vi "Mappatura registri.vi"() -> (3 "Mappa registri":string[][](array[string]))   [LabVIEW 2019]
uses:
  <vilib>/Utility/file.llb/Read From Spreadsheet File (string).vi
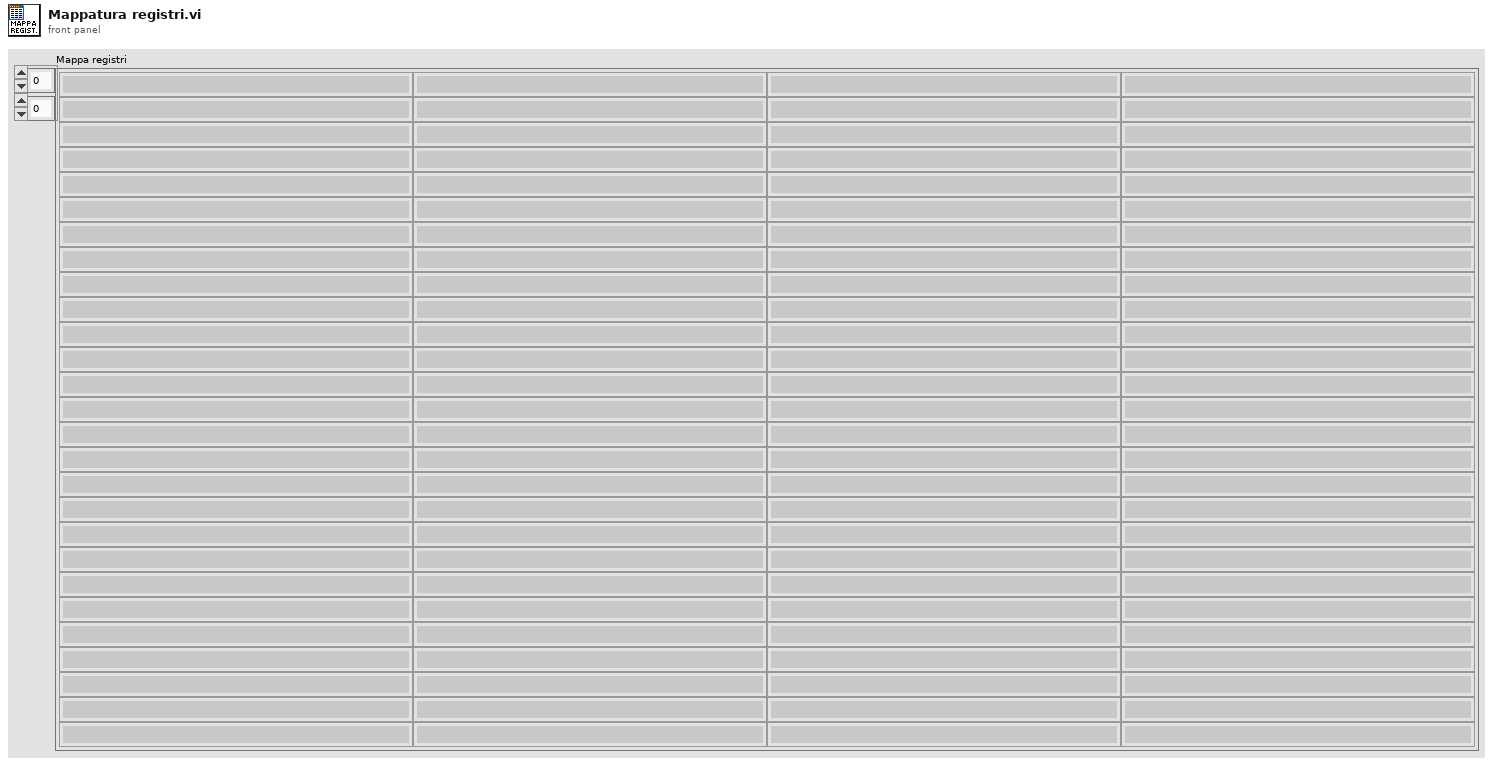
[diagram p1: front panel]
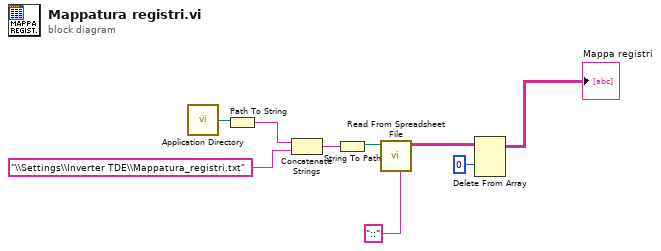
[diagram p0: block diagram]
diagram:
  n1 = call <vilib>:"Application Directory.vi"() -> ("Application Directory"=w5:path)
  n2 = Path To String(path=w5) -> (string=w6:string)
  n3 = Concatenate Strings(w6, "\\Settings\\Inverter TDE\\Mappatura_registri.txt" ("name or relative path")) -> (w8:string)
  n4 = String To Path(string=w8) -> (path=w9:path)
  n5 = call-poly <vilib>:"Read From Spreadsheet File.vi"("delimiter (\\t)"="::" ("delimiter (\\t)"), "file path (dialog if empty)"=w9) -> ("all rows"=w2:string[][])  [unwired: 5 in, 4 out]
  n6 = Delete From Array(array=w2, index (row)=0) -> (array with subset deleted=→"Mappa registri":string[][])  [unwired: 2 in, 1 out]
